vi "Day 1.2 - Calibration value words.vi"(11 "input":string[](array[string])) -> (3 "ouptut part 2":u64)   [LabVIEW 2021]
uses:
  <vilib>/regexp/Match Regular Expression.xnode
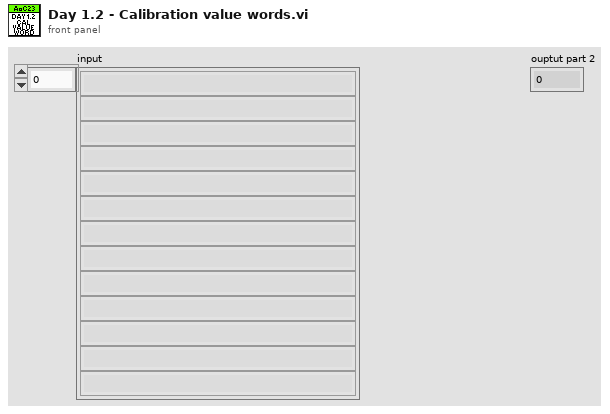
[diagram p1: front panel]
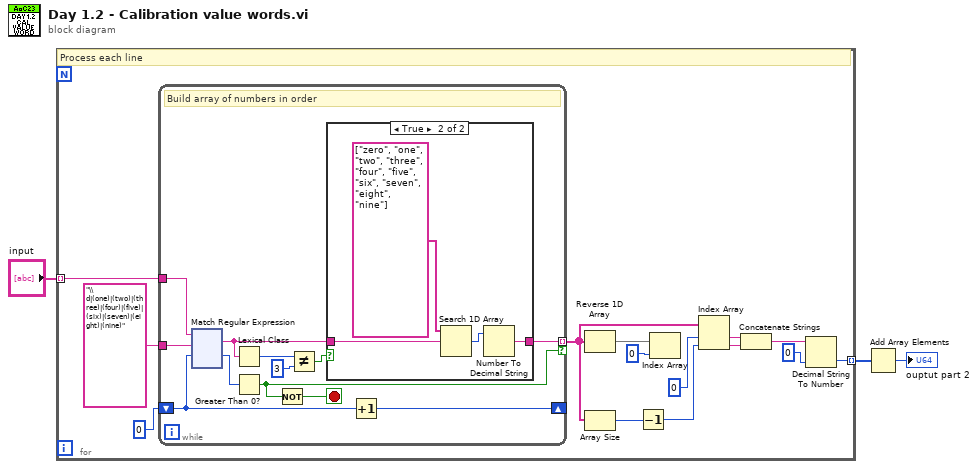
[diagram p0: block diagram]
diagram:
  n1 = for {
    tunnel: "input" -> [w16] mode=indexing
    tunnel: [w17] -> w1 mode=indexing
    # "Process each line"
    n2 = while {
      tunnel: w16 -> [w28]
      tunnel: "\\d|(one)|(two)|(three)|(four)|(five)|(six)|(seven)|(eight)|(nine)" ("regular expression") -> [w27]
      shift-right: [w21] -> _
      shift-left: 0 -> [w23]
      tunnel: [w25] -> w8 mode=indexing if=w24
      stop <- w26 stop-if-true
      # "Build array of numbers in order"
      n3 = xnode "Match Regular Expression"("input string"=w28, "regular expression"=w27, "offset (0)"=w23) -> ("whole match"=w29:string, "offset past match"=w22:i32)  [unwired: 3 in, 3 out]
      n4 = Lexical Class(1:w29) -> (0:w20:i16)
      n5 = Greater Than 0?(x=w22) -> (x > 0?=w24:bool)
      n6 = Not(x=w24) -> (.not. x?=w26:bool)
      n7 = Not Equal?(x=w20, y=i16 3) -> (x != y?=w18:bool)
      n8 = case shown="True" w18 {
        tunnel: w29 -> [w30 w33]
        tunnel: [w30 w32] -> w25
        frame False {
        }
        frame True {
          n9 = Search 1D Array(1D array=string[] ["zero", "one", "two", "three", "four", "five", "six", "seven", "eight", "nine"], element=w33) -> (index of element=w31:i32)  [unwired: 1 in]
          n10 = Number To Decimal String(number=w31) -> (decimal integer string=w32:string)  [unwired: 1 in]
        }
      }
      n11 = Increment(x=w23) -> (x+1=w21:i32)
    }
    n12 = Reverse 1D Array(array=w8) -> (reversed array=w12:string[])
    n13 = Array Size(array=w8) -> (size(s)=w7:i32)
    n14 = Decrement(x=w7) -> (x-1=w5:i32)
    n15 = Index Array(array=w12, index=0) -> ()  [unwired: 1 out]
    n16 = Index Array(array=w8, index #1=0 ("index"), index #2=w5) -> (element #1=w10:string, element #2=w6:string)
    n17 = Concatenate Strings(w10, w6) -> (w4:string)
    n18 = Decimal String To Number(string=w4, default (0L)=u64 0 ("default (0 I32)")) -> (number=w17:u64)  [unwired: 1 in, 1 out]
  }
  n19 = Add Array Elements(numeric array=w1) -> (sum=→"ouptut part 2":u64)
